vi "Clear Trace.vi"(8 "error in (no error)":errorcluster, 10 "Trace  (1: Trace 1)":i32(ring)=1 items=["Trace 1"=1, "Trace 2"=2, "Trace 3"=3, "Trace 4"=4, "Trace 5"=5, "Trace 6"=6, "All"=7], 11 "VISA resource name":refnum<visa-resource-name>) -> (0 "error out":errorcluster, 3 "VISA resource name out":refnum<visa-resource-name>)   [LabVIEW 2014, in "Agilent MXA Series.lvlib"]
doc: "Clears the selected trace."
uses:
  Agilent MXA Series.lvlib
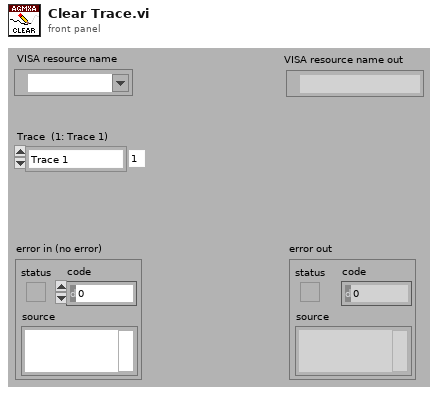
[diagram p1: front panel]
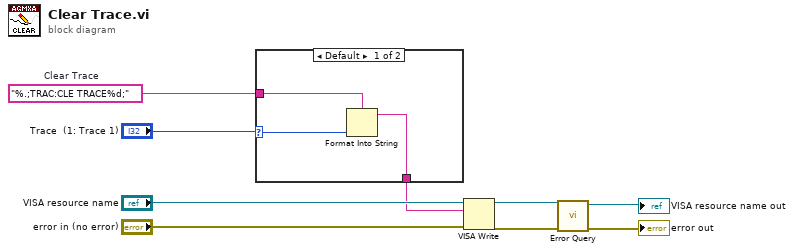
[diagram p0: block diagram]
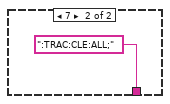
[diagram p2: hidden frame]
diagram:
  w1 = "%.;TRAC:CLE TRACE%d;"  # Clear Trace
  n1 = case shown="Default" "Trace  (1: Trace 1)" {
    selector: "Trace  (1: Trace 1)" -> [w11 _]
    tunnel: [w10 ":TRAC:CLE:ALL;" ("true string")] -> w2
    tunnel: w1 -> [w12 _]
    frame Default {
      n2 = Format Into String(format string=w12, w11) -> (resulting string=w10:string)  [unwired: 2 in, 1 out]
    }
    frame 7 {
    }
  }
  n3 = VISA Write(VISA resource name="VISA resource name", write buffer=w2, error in (no error)="error in (no error)") -> (VISA resource name out=w9:refnum<visa-resource-name>, error out=w6:errorcluster)  [unwired: 1 out]
  n4 = call "Error Query.vi"("error in (no error)"=w6, "VISA resource name"=w9) -> ("error out"=→"error out":errorcluster, "VISA resource name out"=→"VISA resource name out":refnum<visa-resource-name>)  [unwired: 6 in, 2 out]
